vi "Sequence Get Actions.vi"(11 "Excel file in":refnum<class "NI_report.lvclass">) -> (0 "Valid?":bool=TRUE, 2 "Actions":T1[](array[typedef]))   [LabVIEW 2015]
uses:
  <vilib>/Utility/NIReport.llb/NI_report.lvclass
  Test Sequence Action.ctl
  Valve Action Enum.ctl
  Valve Name Enum.ctl
  <vilib>/addons/_office/excel.llb/Excel Get Data ([str]).vi
  <vilib>/addons/_office/NI_ReportGenerationToolkit.lvlib
  <vilib>/Utility/NIReport.llb/Excel/NI_Excel.lvclass
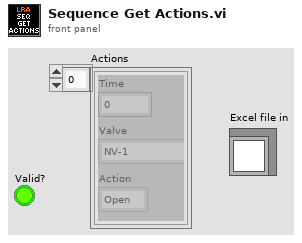
[diagram p1: front panel]
types:
  T1 = typedef "Test Sequence Action.ctl" = cluster{"Time":i32, "Action":T2, "Valve":T3}
  T2 = typedef "Valve Action Enum.ctl" = enum16{"Open", "Close"}
  T3 = typedef "Valve Name Enum.ctl" = enum16{"NV-1", "NV-2", "OV-2", "OV-3", "OV-4", "WV-2"}
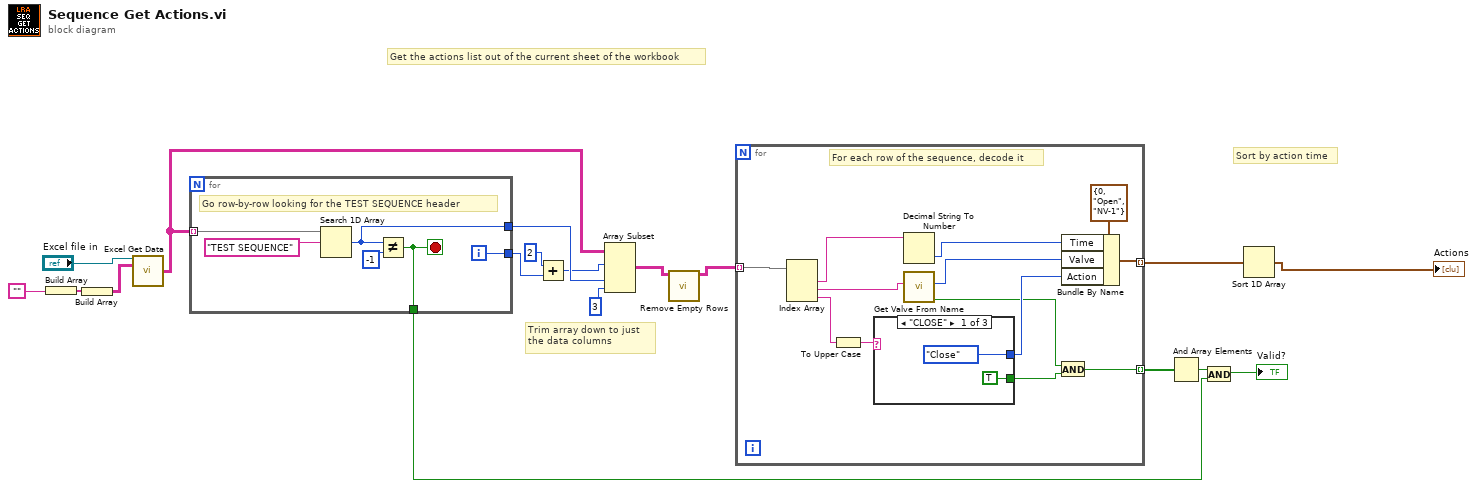
[diagram p0: block diagram]
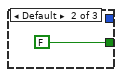
[diagram p2: hidden frame]
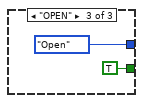
[diagram p3: hidden frame]
diagram:
  # "Sort by action time"
  # "Trim array down to just \nthe data columns"
  # "Get the actions list out of the current sheet of the workbook"
  n1 = Build Array("") -> (w16:string[])
  n2 = Build Array(w16) -> (w15:string[][])
  n3 = call-poly <vilib>:"Excel Get Data.vi"("report in"="Excel file in", "data type"=w15) -> ("data"=w14:string[][])  [unwired: 11 in, 2 out]
  n4 = for {
    tunnel: w14 -> [w24] mode=indexing
    tunnel: [w21] -> w12
    tunnel: [w20] -> w10
    tunnel: [w19] -> w5
    i -> [w20]
    stop <- w19 stop-if-true
    # "Go row-by-row looking for the TEST SEQUENCE header"
    n5 = Search 1D Array(1D array=w24, element="TEST SEQUENCE") -> (index of element=w21:i32)  [unwired: 1 in]
    n6 = Not Equal?(x=w21, y=-1) -> (x != y?=w19:bool)
  }
  n7 = Add(x=2, y=w10) -> (x+y=w9:i32)
  n8 = Array Subset(array=w14, index (row)=w9, index (col)=w12, length (col)=3 ("length")) -> (w4:string[][])  [unwired: 1 in]
  n9 = call "Remove Empty Rows.vi"("Array in"=w4) -> ("Array out"=w3:string[][])  [unwired: 10 in]
  n10 = for {
    tunnel: w3 -> [w35] mode=indexing
    tunnel: [w36] -> w2 mode=indexing
    tunnel: [w25] -> w8 mode=indexing
    # "For each row of the sequence, decode it"
    n11 = Index Array(array=w35) -> (element #1=w34:string, element #2=w32:string, element #3=w30:string)  [unwired: 3 in]
    n12 = To Upper Case(1:w30) -> (0:w29:string)
    n13 = case shown="\"CLOSE\"" w29 {
      tunnel: [Valve_Action_Enum."Close" ("Action") _ Valve_Action_Enum."Open" ("Action")] -> w28
      tunnel: [TRUE FALSE TRUE] -> w27
      frame "CLOSE" {
      }
      frame Default {
      }
      frame "OPEN" {
      }
    }
    n14 = Decimal String To Number(string=w34) -> (number=w33:i32)  [unwired: 2 in, 1 out]
    n15 = call "Get Valve From Name.vi"("Name"=w32) -> ("Valid?"=w26:bool, "Valve"=w31:T3)  [unwired: 9 in]
    n16 = And(x=w26, y=w27) -> (x .and. y?=w25:bool)
    n17 = Bundle By Name(cluster=T1 {"Time"=0, "Action"=enum."Open", "Valve"=enum."NV-1"} ("input cluster"), "Time"=w33, "Valve"=w31, "Action"=w28) -> (w36:T1)
  }
  n18 = And Array Elements(Boolean array=w8) -> (logical AND=w7:bool)
  n19 = And(x=w7, y=w5) -> (x .and. y?=→"Valid?":bool)
  n20 = Sort 1D Array(array=w2) -> (sorted array=→"Actions":T1[])
